vi "Dialog.vi"(7 "Language":T1, 11 "Message":string caption="Test file exists. Do you want to overwrite the data?") -> (3 "Exit?":bool)   [LabVIEW 2024]
uses:
  Controls/Language.ctl
  <vilib>/addons/Tools/Unicode/UI Unicode Tools.lvlib
panel:
  in  "OK Button":bool
  in  "Cancel Button":bool
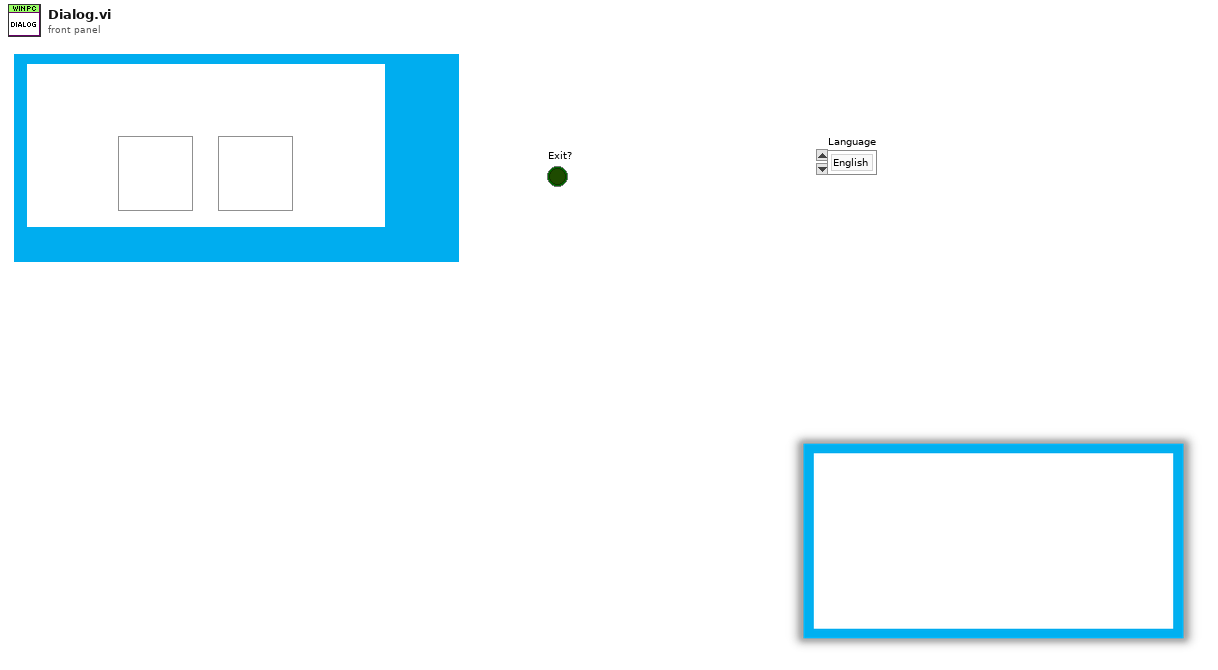
[diagram p1: front panel]
types:
  T1 = typedef "Language.ctl" = enum16{"English", "Chinese", "German"}
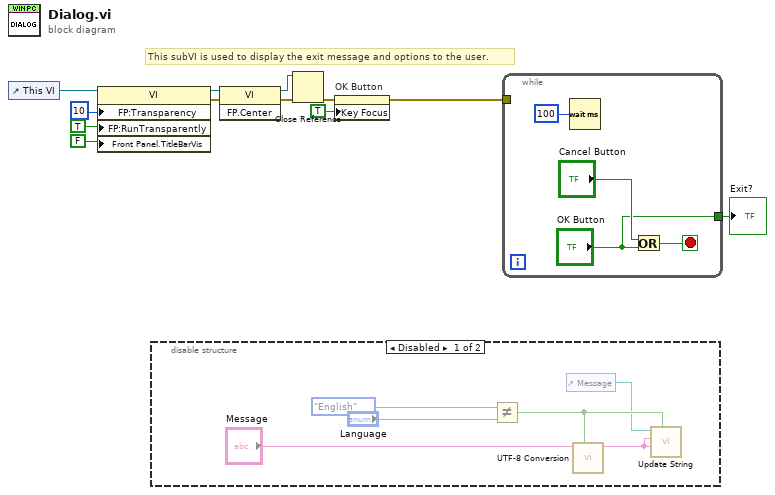
[diagram p0: block diagram]
diagram:
  # "This subVI is used to display the exit message and options to the user."
  n1 = control-ref of="This VI"() -> (w10:refnum<vi>)
  n2 = property class="VI"(reference=w10, "FP:Transparency"=u8 10 ("Front Panel Window:Transparency"), "FP:RunTransparently"=TRUE ("Front Panel Window:Title Bar Visible"), "Front Panel.TitleBarVis"=FALSE ("Front Panel Window:Title Bar Visible")) -> (reference out=w8:refnum<vi>, error out=w7:errorcluster)  [unwired: 1 in]
  n3 = disable-structure shown="Disabled" {
    frame Disabled {
      n4 = Not Equal?(x=Language."English" ("UI Information.Language"), y="Language") -> (x != y?=w15:bool)
      n5 = control-ref of="Message"() -> (w14:refnum<vi>)
      n6 = call "UTF-8 Conversion.vi"("Unicode?"=w15, "Config String"="Message") -> ("Unicode/ANSI string"=w18:string)  [unwired: 8 in, 1 out]
      n7 = call <vilib>:"Update String.vi"("Interpret as Unicode (T)"=w15, "Caption"=w18, "String Value"=w18, "String Control Reference"=w14) -> ()  [unwired: 4 in, 2 out]
    }
    frame Enabled {
    }
  }
  n8 = invoke class="VI" method="FP.Center"(reference=w8, error in=w7) -> (reference out=w12:refnum<vi>, error out=w11:errorcluster)  [unwired: 1 in, 1 out]
  n9 = Close Reference(reference=w12, error in (no error)=w11) -> (error out=w2:errorcluster)
  n10 = property on="OK Button" class="Bool"(error in=w2, "Key Focus"=TRUE) -> (error out=w1:errorcluster)  [unwired: 1 in, 1 out]
  n11 = while {
    tunnel: ["OK Button"] -> w4
    tunnel: w1 -> [_]
    stop <- w21 stop-if-true
    n12 = Wait (ms)(milliseconds to wait=u32 100) -> ()  [unwired: 1 out]
    n13 = Or(x="Cancel Button", y="OK Button") -> (x .or. y?=w21:bool)
  }
  "Exit?" <- w4
